vi "UNBILITZ-ShutterDriver-Open.vi"(0 "VISA resource name":refnum<visa-resource-name>, 2 "Simulation Mode?":bool, 11 "error in (no error)":errorcluster) -> (4 "VISA resource name out":refnum<visa-resource-name>, 15 "error out":errorcluster)   [LabVIEW 2013]
doc: "Opens a serial connection to the Uniblitz shutter driver (this terminology is used by Uniblitz to describe the hardware device which controls their shutters; it is this device with which this software driver communicates)."
uses:
  <vilib>/Instr/_visa.llb/VISA Configure Serial Port (Instr).vi
  UNIBLITZ-SimulationModeOperation.ctl
panel:
  # "Inputs"
  # "Outputs"
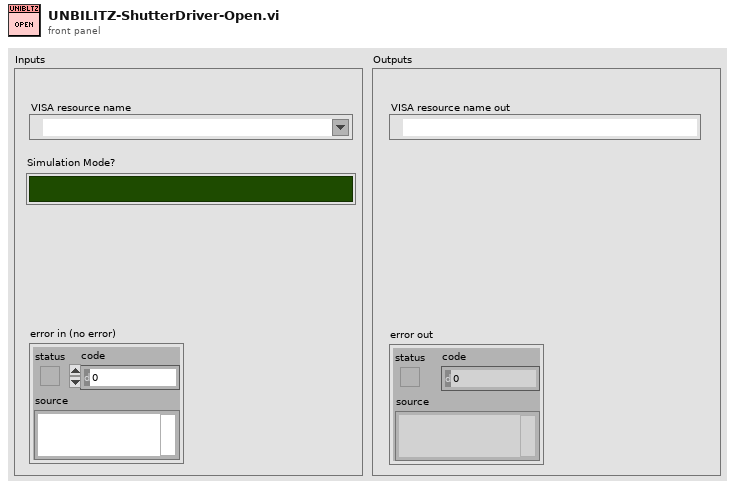
[diagram p1: front panel]
types:
  T1 = typedef "UNIBLITZ-SimulationModeOperation.ctl" = enum16{"Get", "Set"}
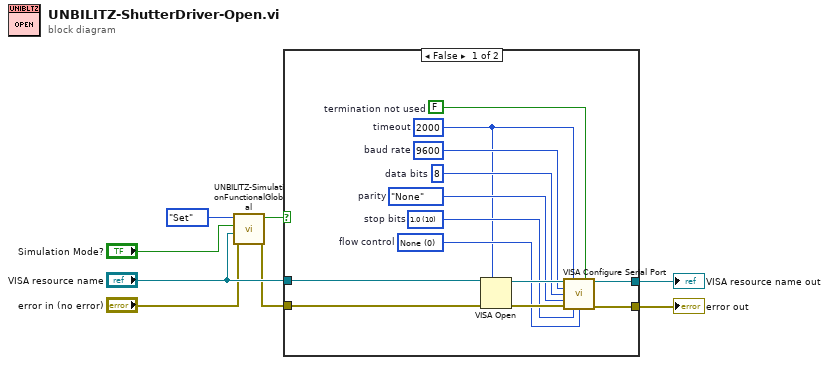
[diagram p0: block diagram]
diagram:
  n1 = call "UNBILITZ-SimulationFunctionalGlobal.vi"("error in (no error)"="error in (no error)", "VISA Resource Name"="VISA resource name", "Simulation Mode"="Simulation Mode?", "Operation (Get)"=UNIBLITZ-SimulationModeOperation."Set") -> ("error out"=w2:errorcluster, "Simulation Mode"=w1:bool)  [unwired: 6 in]
  n2 = case shown="False" w1 {
    tunnel: [w19 w23] -> w8
    tunnel: [w18 w22] -> w7
    tunnel: "VISA resource name" -> [w10 w23]
    tunnel: w2 -> [w9 w22]
    frame False {
      w12 = u16 0 items=["None", "XON/XOFF", "RTS/CTS", "XON/XOFF & RTS/CTS", "DTR/DSR", "XON/XOFF & DTR/DSR"]  # flow control
      w13 = u16 10 items=["1.0"=10, "1.5"=15, "2.0"=20]  # stop bits
      w14 = enum16{"None", "Odd", "Even", "Mark", "Space"}."None"  # parity
      w15 = u16 8  # data bits
      w16 = u32 9600  # baud rate
      w17 = FALSE  # termination not used
      w11 = u32 2000  # timeout
      n3 = VISA Open(timeout (0)=w11, error in (no error)=w9, VISA resource name=w10) -> (VISA resource name=w21:refnum<visa-resource-name>, error out=w20:errorcluster)  [unwired: 2 in]
      n4 = call-poly "VISA Configure Serial Port"("VISA resource name"=w21, "timeout (10sec)"=w11, "Enable Termination\nChar (T)"=w17, "baud rate (9600)"=w16, "data bits (8)"=w15, "parity (0:none)"=w14, "error in (no error)"=w20, "stop bits (10: 1 bit)"=w13, "flow control (0:none)"=w12) -> ("VISA resource name out"=w19:refnum<visa-resource-name>, "error out"=w18:errorcluster)  [unwired: 5 in]
    }
    frame True {
    }
  }
  "error out" <- w7
  "VISA resource name out" <- w8
